vi "Get Random.vi"(7 "Func_Ext":string, 8 "에러 입력":errorcluster caption="에러 입력(에러 없음)", 10 "분해능":string caption="분해능(우선적용)", 11 "Meas":refnum<vi>[](array[refnum])) -> (0 "에러 출력":errorcluster, 3 "Meas out":refnum<vi>[](array[refnum]))   [LabVIEW 2020]
uses:
  Controls/Cmd_Var Data IO.ctl
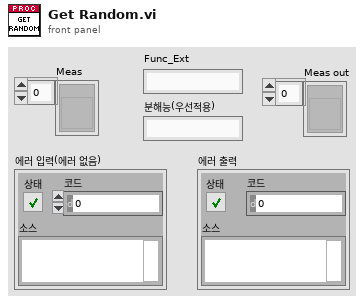
[diagram p1: front panel]
types:
  T1 = typedef "Cmd_Var Data IO.ctl" = enum16{"Condition", "Condition Default", "Condition_Temp", "Resolution", "Resolution Default", "Resolution Old", "Spec", "Spec Default", "Spec Old", "Spec Temp", "Result", "Result2", "Result3", "Result_Temp", "Result_ADJ", "Result_ADJ2", "STD1", "STD2", "STD3", "STD4", "STD5", "STD Temp", "CMC", "CMC Default"}
  T2 = enum8{"Enabled", "Disabled", "Disabled and Grayed Out"}
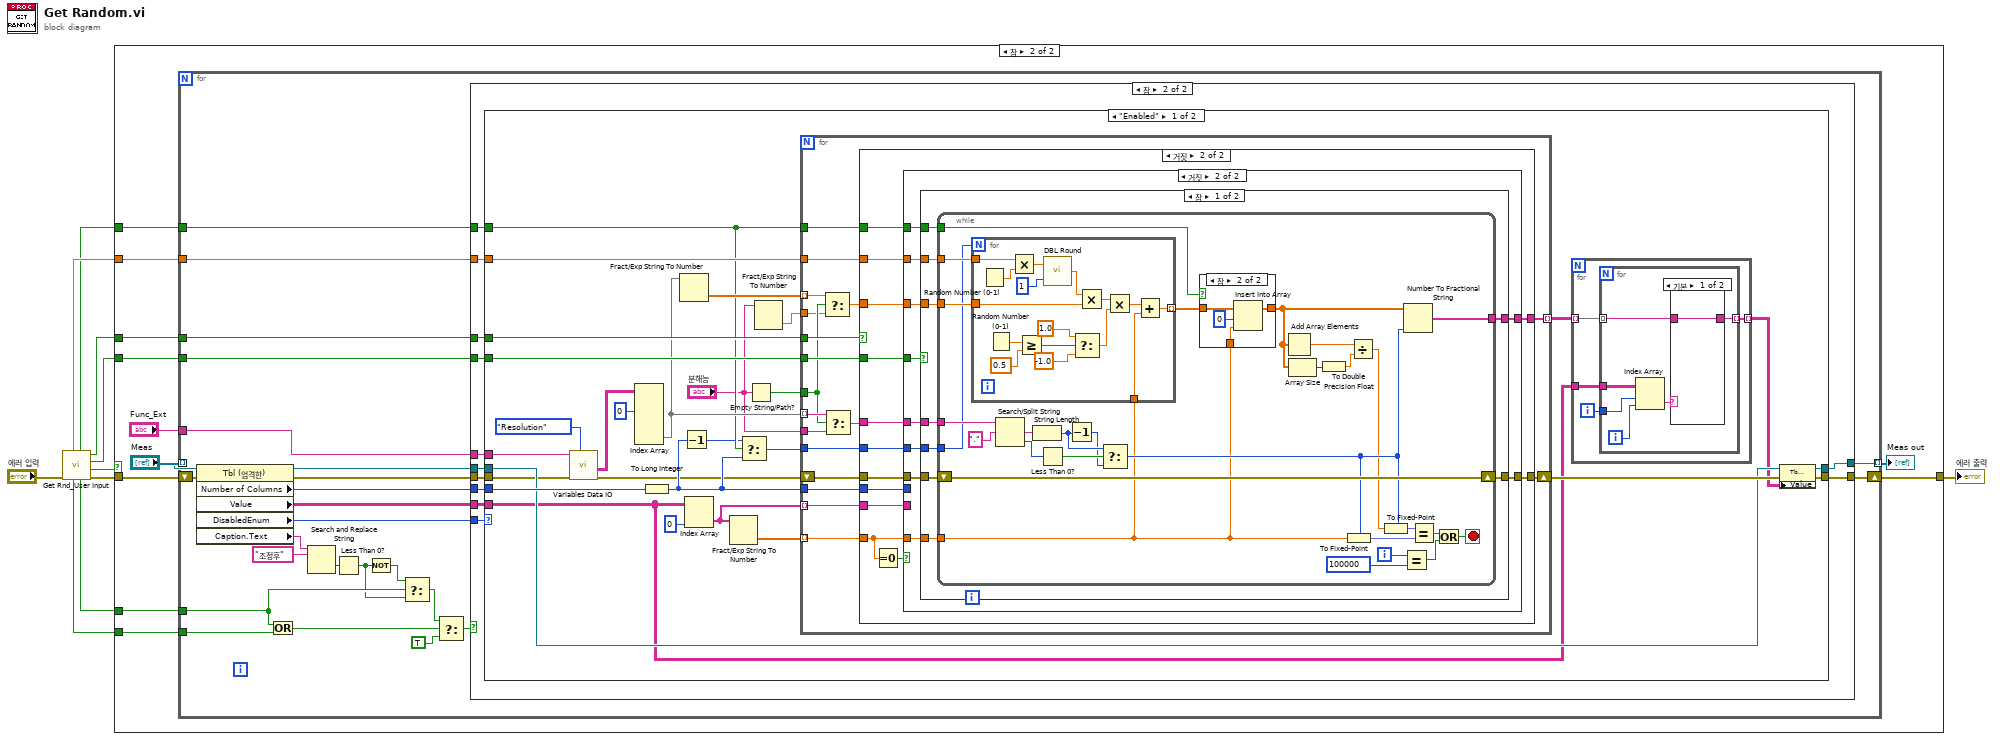
[diagram p0: block diagram]
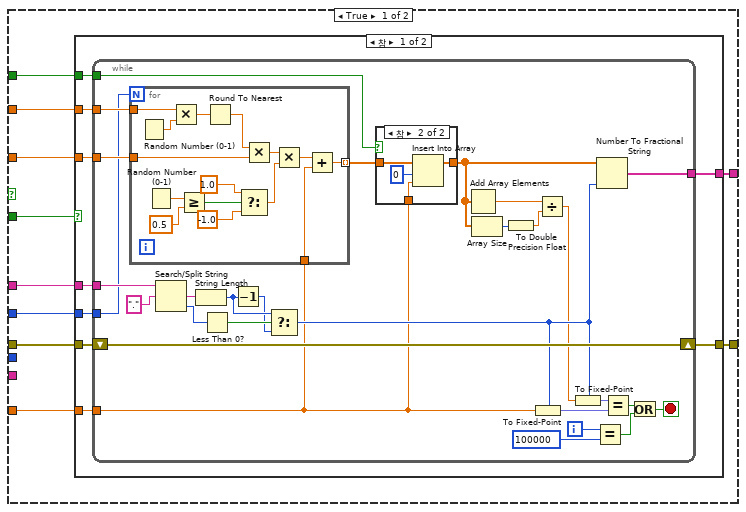
[diagram p5: hidden frame]
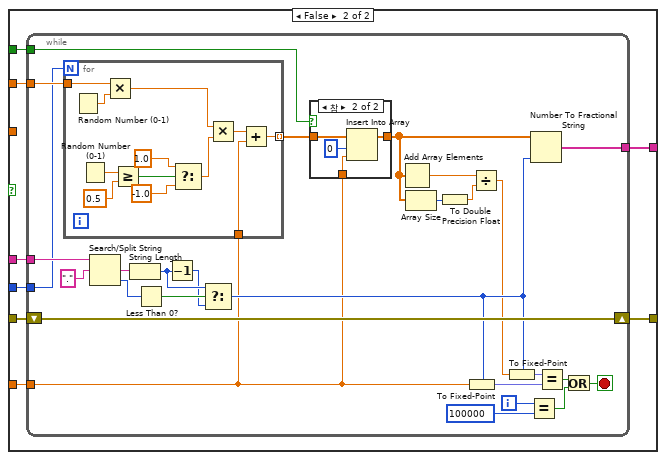
[diagram p7: hidden frame]
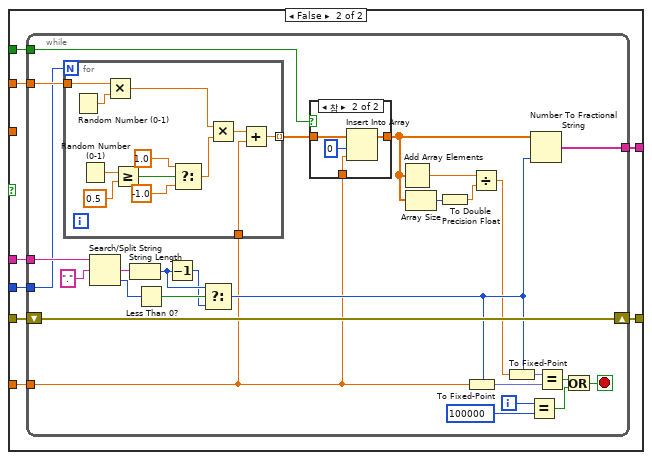
[diagram p11: hidden frame]
diagram:
  n1 = call "Get Rnd_User Input.vi"("error in"="에러 입력") -> ("error out"=w8:errorcluster, "변경?"=w7:bool, "분해능 기준?"=w4:bool, "0점 포함?"=w5:bool, "조정후?"=w1:bool, "1열 제외?"=w3:bool, "조정전?"=w2:bool, "변화량"=w6:dbl)  [unwired: 3 in]
  n2 = case shown="참" w7 {
    tunnel: [w11 w22] -> w10
    tunnel: w8 -> [w11 w19]
    tunnel: w6 -> [_ w18]
    tunnel: w5 -> [_ w17]
    tunnel: w4 -> [_ w16]
    tunnel: w3 -> [_ w15]
    tunnel: w2 -> [_ w13]
    tunnel: w1 -> [_ w12]
    frame False {
    }
    frame True {
      n3 = for {
        tunnel: "Meas" -> [w47] mode=indexing
        shift-right: [w44] -> w22
        shift-left: w19 -> [w37]
        tunnel: "Func_Ext" -> [w40]
        tunnel: w18 -> [w45]
        tunnel: w17 -> [w42]
        tunnel: w16 -> [w41]
        tunnel: w15 -> [w39]
        tunnel: [w34] -> w14 mode=indexing
        tunnel: w13 -> [w30]
        tunnel: w12 -> [w26]
        n4 = property on="프로퍼티 노드" class="Tbl (엄격한)"(reference=w47, error in=w37) -> (reference out=w43:refnum<vi>, error out=w36:errorcluster, "Number of Columns"=w46:u32, "Value"=w38:string[][], "DisabledEnum"=w35:T2, "Caption.Text"=w33:string)
        n5 = Or(x=w26, y=w30) -> (x .or. y?=w28:bool)
        n6 = Search and Replace String(input string=w33, search string="조정후" ("검색 문자열")) -> (offset past replacement=w27:i32)  [unwired: 6 in, 3 out]
        n7 = Less Than 0?(x=w27) -> (x < 0?=w24:bool)
        n8 = Not(x=w24) -> (.not. x?=w23:bool)
        n9 = Select(t=w23, s=w26, f=w24) -> (s? t:f=w25:bool)
        n10 = Select(t=w25, s=w28, f=TRUE) -> (s? t:f=w31:bool)
        n11 = case shown="참" w31 {
          tunnel: w46 -> [_ w61]
          tunnel: w45 -> [_ w60]
          tunnel: [w48 w59] -> w44
          tunnel: w43 -> [w49 w58]
          tunnel: w42 -> [_ w57]
          tunnel: w41 -> [_ w56]
          tunnel: w40 -> [_ w55]
          tunnel: w39 -> [_ w54]
          tunnel: w38 -> [_ w53]
          tunnel: w36 -> [w48 w52]
          tunnel: w35 -> [_ w51]
          tunnel: [w49 w50] -> w34
          frame False {
          }
          frame True {
            n12 = case shown="\"Enabled\"" w51 {
              tunnel: w61 -> [w89 _]
              tunnel: w60 -> [w83 _]
              tunnel: [w81 w379] -> w59
              tunnel: w58 -> [w80 w378]
              tunnel: w57 -> [w79 _]
              tunnel: w56 -> [w77 _]
              tunnel: w55 -> [w75 _]
              tunnel: w54 -> [w74 _]
              tunnel: w53 -> [w67 _]
              tunnel: w52 -> [w64 w379]
              tunnel: [w62 w378] -> w50
              frame "Enabled" {
                n13 = call "Variables Data IO.vi"("Select"=Cmd_Var_Data_IO."Resolution", "error in"=w64, "Func_ext"=w75) -> ("error out"=w63:errorcluster, "Data Out"=w86:string[][])  [unwired: 6 in, 1 out]
                n14 = Index Array(array=w86, index (col) #1=0 ("비활성화된 인덱스 (열)")) -> (element #3=w76:string[])  [unwired: 5 in, 2 out]
                n15 = To Long Integer(number=w89) -> (32bit integer=w72:i32)
                n16 = Fract/Exp String To Number(string=w76) -> (number=w85:dbl[])  [unwired: 3 in, 1 out]
                n17 = Decrement(x=w72) -> (x-1=w73:i32)
                n18 = Index Array(array=w67, index (col)=0 ("비활성화된 인덱스 (열)")) -> (element=w78:string[])  [unwired: 1 in]
                n19 = Fract/Exp String To Number(string=w78) -> (number=w88:dbl[])  [unwired: 3 in, 1 out]
                n20 = Select(t=w73, s=w74, f=w72) -> (s? t:f=w71:i32)
                n21 = Empty String/Path?(string/path="분해능") -> (empty?=w70:bool)
                n22 = Fract/Exp String To Number(string="분해능") -> (number=w68:dbl)  [unwired: 3 in, 1 out]
                n23 = for {
                  tunnel: w88 -> [w119] mode=indexing
                  tunnel: w72 -> [w120]
                  shift-right: [w117] -> w82
                  shift-left: w63 -> [w118]
                  tunnel: w85 -> [w105] mode=indexing
                  tunnel: w76 -> [w109] mode=indexing
                  tunnel: w83 -> [w116]
                  tunnel: [w115] -> w66 mode=indexing
                  tunnel: w79 -> [w114]
                  tunnel: w78 -> [w113] mode=indexing
                  tunnel: w77 -> [w112]
                  tunnel: w74 -> [w111]
                  tunnel: w71 -> [w110]
                  tunnel: w70 -> [w104]
                  tunnel: "분해능" -> [w107]
                  tunnel: w68 -> [w103]
                  n24 = Select(t=w105, s=w104, f=w103) -> (s? t:f=w106:dbl)
                  n25 = Select(t=w109, s=w104, f=w107) -> (s? t:f=w108:string)
                  n26 = case shown="거짓" w114 {
                    tunnel: w120 -> [_ w252]
                    tunnel: w119 -> [w123 w243]
                    tunnel: w106 -> [w127 w246]
                    tunnel: w108 -> [w125 w251]
                    tunnel: w118 -> [w124 w250]
                    tunnel: [w129 w249] -> w117
                    tunnel: w116 -> [w128 w248]
                    tunnel: [w130 w247] -> w115
                    tunnel: w113 -> [_ w244]
                    tunnel: w112 -> [w126 w242]
                    tunnel: w111 -> [w121 w241]
                    tunnel: w110 -> [w122 w240]
                    frame True {
                      n27 = case shown="참" w126 {
                        tunnel: w123 -> [w139 w195]
                        tunnel: w127 -> [w138 _]
                        tunnel: w125 -> [w137 w194]
                        tunnel: w124 -> [w136 w193]
                        tunnel: [w135 w192] -> w129
                        tunnel: w128 -> [w134 w191]
                        tunnel: [w133 w190] -> w130
                        tunnel: w122 -> [w132 w189]
                        tunnel: w121 -> [w131 w188]
                        frame True {
                          n28 = while {
                            tunnel: w139 -> [w143]
                            tunnel: w138 -> [w167]
                            tunnel: w137 -> [w166]
                            shift-right: [w163] -> w135
                            shift-left: w136 -> [w163]
                            tunnel: w134 -> [w151]
                            tunnel: [w149] -> w133
                            tunnel: w132 -> [w144]
                            tunnel: w131 -> [w140]
                            i -> [w165]
                            stop <- w158 stop-if-true
                            n29 = for {
                              N: w144 -> [_]
                              tunnel: w143 -> [w180]
                              tunnel: w167 -> [w178]
                              tunnel: [w179] -> w141 mode=indexing
                              tunnel: w151 -> [w174]
                              n30 = Random Number (0-1)() -> (number: 0 to 1=w175:dbl)
                              n31 = Random Number (0-1)() -> (number: 0 to 1=w187:dbl)
                              n32 = Multiply(x=w174, y=w175) -> (x*y=w176:dbl)
                              n33 = Greater Or Equal?(x=w187, y=0.5) -> (x >= y?=w185:bool)
                              n34 = Round To Nearest(number=w176) -> (nearest integer value=w173:dbl)
                              n35 = Select(t=1.0, s=w185, f=-1.0) -> (s? t:f=w182:dbl)
                              n36 = Multiply(x=w173, y=w178) -> (x*y=w177:dbl)
                              n37 = Multiply(x=w177, y=w182) -> (x*y=w181:dbl)
                              n38 = Add(x=w181, y=w180) -> (x+y=w179:dbl)
                            }
                            n39 = Search/Split String(string=w166, search string/char (-)="." ("검색 문자열/문자 (-)")) -> (match + rest of string=w157:string, offset of match=w155:i32)  [unwired: 1 in, 1 out]
                            n40 = String Length(string=w157) -> (length=w153:i32)
                            n41 = Less Than 0?(x=w155) -> (x < 0?=w154:bool)
                            n42 = Decrement(x=w153) -> (x-1=w152:i32)
                            n43 = Select(t=w153, s=w154, f=w152) -> (s? t:f=w150:i32)
                            n44 = case shown="참" w140 {
                              tunnel: w141 -> [w168 w172]
                              tunnel: w143 -> [_ w170]
                              tunnel: [w168 w169] -> w142
                              frame False {
                              }
                              frame True {
                                n45 = Insert Into Array(array=w172, index=0 ("인덱스"), new element=w170) -> (w169:dbl[])
                              }
                            }
                            n46 = Add Array Elements(numeric array=w142) -> (sum=w148:dbl)
                            n47 = Array Size(array=w142) -> (size(s)=w147:i32)
                            n48 = To Double Precision Float(number=w147) -> (double precision float=w146:dbl)
                            n49 = To Fixed-Point(fixed-point type=w150, number=w143) -> (fixed-point=w161:fxp<+/-,32,32>)
                            n50 = Divide(x=w148, y=w146) -> (x/y=w145:dbl)
                            n51 = To Fixed-Point(fixed-point type=w150, number=w145) -> (fixed-point=w162:fxp<+/-,32,32>)
                            n52 = Equal?(x=w165, y=100000) -> (x = y?=w159:bool)
                            n53 = Number To Fractional String(number=w142, precision (6)=w150) -> (F-format string=w149:string[])  [unwired: 2 in]
                            n54 = Equal?(x=w162, y=w161) -> (x = y?=w160:bool)
                            n55 = Or(x=w160, y=w159) -> (x .or. y?=w158:bool)
                          }
                        }
                        frame False {
                          n56 = while {
                            tunnel: w195 -> [w203]
                            tunnel: w194 -> [w222]
                            shift-right: [w219] -> w192
                            shift-left: w193 -> [w219]
                            tunnel: w191 -> [w207]
                            tunnel: [w204] -> w190
                            tunnel: w189 -> [w197]
                            tunnel: w188 -> [w196]
                            i -> [w221]
                            stop <- w214 stop-if-true
                            n57 = for {
                              N: w197 -> [_]
                              tunnel: w203 -> [w238]
                              tunnel: [w237] -> w206 mode=indexing
                              tunnel: w207 -> [w229]
                              n58 = Random Number (0-1)() -> (number: 0 to 1=w236:dbl)
                              n59 = Random Number (0-1)() -> (number: 0 to 1=w235:dbl)
                              n60 = Multiply(x=w229, y=w236) -> (x*y=w228:dbl)
                              n61 = Greater Or Equal?(x=w235, y=0.5) -> (x >= y?=w234:bool)
                              n62 = Select(t=1.0, s=w234, f=-1.0) -> (s? t:f=w232:dbl)
                              n63 = Multiply(x=w228, y=w232) -> (x*y=w239:dbl)
                              n64 = Add(x=w239, y=w238) -> (x+y=w237:dbl)
                            }
                            n65 = Search/Split String(string=w222, search string/char (-)="." ("검색 문자열/문자 (-)")) -> (match + rest of string=w213:string, offset of match=w211:i32)  [unwired: 1 in, 1 out]
                            n66 = String Length(string=w213) -> (length=w209:i32)
                            n67 = Less Than 0?(x=w211) -> (x < 0?=w210:bool)
                            n68 = Decrement(x=w209) -> (x-1=w208:i32)
                            n69 = Select(t=w209, s=w210, f=w208) -> (s? t:f=w205:i32)
                            n70 = case shown="참" w196 {
                              tunnel: w206 -> [w223 w227]
                              tunnel: w203 -> [_ w225]
                              tunnel: [w223 w224] -> w199
                              frame False {
                              }
                              frame True {
                                n71 = Insert Into Array(array=w227, index=0 ("인덱스"), new element=w225) -> (w224:dbl[])
                              }
                            }
                            n72 = Add Array Elements(numeric array=w199) -> (sum=w202:dbl)
                            n73 = Array Size(array=w199) -> (size(s)=w201:i32)
                            n74 = To Double Precision Float(number=w201) -> (double precision float=w200:dbl)
                            n75 = To Fixed-Point(fixed-point type=w205, number=w203) -> (fixed-point=w217:fxp<+/-,32,32>)
                            n76 = Divide(x=w202, y=w200) -> (x/y=w198:dbl)
                            n77 = To Fixed-Point(fixed-point type=w205, number=w198) -> (fixed-point=w218:fxp<+/-,32,32>)
                            n78 = Equal?(x=w221, y=100000) -> (x = y?=w215:bool)
                            n79 = Number To Fractional String(number=w199, precision (6)=w205) -> (F-format string=w204:string[])  [unwired: 2 in]
                            n80 = Equal?(x=w218, y=w217) -> (x = y?=w216:bool)
                            n81 = Or(x=w216, y=w215) -> (x .or. y?=w214:bool)
                          }
                        }
                      }
                    }
                    frame False {
                      n82 = Equal To 0?(x=w243) -> (x = 0?=w245:bool)
                      n83 = case shown="거짓" w245 {
                        tunnel: w252 -> [w255 _]
                        tunnel: w243 -> [_ w267]
                        tunnel: w246 -> [_ w266]
                        tunnel: w251 -> [_ w265]
                        tunnel: w250 -> [w256 w264]
                        tunnel: [w256 w263] -> w249
                        tunnel: w248 -> [_ w262]
                        tunnel: [w254 w261] -> w247
                        tunnel: w244 -> [w253 _]
                        tunnel: w242 -> [_ w260]
                        tunnel: w241 -> [_ w259]
                        tunnel: w240 -> [_ w258]
                        frame True {
                          n84 = for {
                            N: w255 -> [_]
                            tunnel: w253 -> [w257]
                            tunnel: [w257] -> w254 mode=indexing
                          }
                        }
                        frame False {
                          n85 = case shown="참" w260 {
                            tunnel: w267 -> [w276 w333]
                            tunnel: w266 -> [w275 _]
                            tunnel: w265 -> [w274 w332]
                            tunnel: w264 -> [w273 w331]
                            tunnel: [w272 w330] -> w263
                            tunnel: w262 -> [w271 w329]
                            tunnel: [w270 w328] -> w261
                            tunnel: w259 -> [w269 w326]
                            tunnel: w258 -> [w268 w327]
                            frame True {
                              n86 = while {
                                tunnel: w276 -> [w279]
                                tunnel: w275 -> [w304]
                                tunnel: w274 -> [w303]
                                shift-right: [w300] -> w272
                                shift-left: w273 -> [w300]
                                tunnel: w271 -> [w288]
                                tunnel: [w286] -> w270
                                tunnel: w269 -> [w277]
                                tunnel: w268 -> [w281]
                                i -> [w302]
                                stop <- w295 stop-if-true
                                n87 = for {
                                N: w281 -> [_]
                                tunnel: w279 -> [w318]
                                tunnel: w304 -> [w314]
                                tunnel: [w317] -> w280 mode=indexing
                                tunnel: w288 -> [w315]
                                n88 = Random Number (0-1)() -> (number: 0 to 1=w316:dbl)
                                n89 = Random Number (0-1)() -> (number: 0 to 1=w325:dbl)
                                n90 = Multiply(x=w315, y=w316) -> (x*y=w312:dbl)
                                n91 = Greater Or Equal?(x=w325, y=0.5) -> (x >= y?=w323:bool)
                                n92 = call "DBL Round.vi"("반올림자리수"=1 ("자리수"), "DBL in"=w312) -> ("DBL out"=w311:dbl)  [unwired: 1 in]
                                n93 = Select(t=1.0, s=w323, f=-1.0) -> (s? t:f=w320:dbl)
                                n94 = Multiply(x=w311, y=w314) -> (x*y=w313:dbl)
                                n95 = Multiply(x=w313, y=w320) -> (x*y=w319:dbl)
                                n96 = Add(x=w319, y=w318) -> (x+y=w317:dbl)
                                }
                                n97 = Search/Split String(string=w303, search string/char (-)="." ("검색 문자열/문자 (-)")) -> (match + rest of string=w294:string, offset of match=w292:i32)  [unwired: 1 in, 1 out]
                                n98 = String Length(string=w294) -> (length=w290:i32)
                                n99 = Less Than 0?(x=w292) -> (x < 0?=w291:bool)
                                n100 = Decrement(x=w290) -> (x-1=w289:i32)
                                n101 = Select(t=w290, s=w291, f=w289) -> (s? t:f=w287:i32)
                                n102 = case shown="참" w277 {
                                tunnel: w280 -> [w305 w309]
                                tunnel: w279 -> [_ w307]
                                tunnel: [w305 w306] -> w278
                                frame False {
                                }
                                frame True {
                                n103 = Insert Into Array(array=w309, index=0 ("인덱스"), new element=w307) -> (w306:dbl[])
                                }
                                }
                                n104 = Add Array Elements(numeric array=w278) -> (sum=w285:dbl)
                                n105 = Array Size(array=w278) -> (size(s)=w284:i32)
                                n106 = To Double Precision Float(number=w284) -> (double precision float=w283:dbl)
                                n107 = To Fixed-Point(fixed-point type=w287, number=w279) -> (fixed-point=w298:fxp<+/-,32,32>)
                                n108 = Divide(x=w285, y=w283) -> (x/y=w282:dbl)
                                n109 = To Fixed-Point(fixed-point type=w287, number=w282) -> (fixed-point=w299:fxp<+/-,32,32>)
                                n110 = Equal?(x=w302, y=100000) -> (x = y?=w296:bool)
                                n111 = Number To Fractional String(number=w278, precision (6)=w287) -> (F-format string=w286:string[])  [unwired: 2 in]
                                n112 = Equal?(x=w299, y=w298) -> (x = y?=w297:bool)
                                n113 = Or(x=w297, y=w296) -> (x .or. y?=w295:bool)
                              }
                            }
                            frame False {
                              n114 = while {
                                tunnel: w333 -> [w336]
                                tunnel: w332 -> [w360]
                                shift-right: [w357] -> w330
                                shift-left: w331 -> [w357]
                                tunnel: w329 -> [w345]
                                tunnel: [w343] -> w328
                                tunnel: w327 -> [w338]
                                tunnel: w326 -> [w334]
                                i -> [w359]
                                stop <- w352 stop-if-true
                                n115 = for {
                                N: w338 -> [_]
                                tunnel: w336 -> [w376]
                                tunnel: [w375] -> w337 mode=indexing
                                tunnel: w345 -> [w367]
                                n116 = Random Number (0-1)() -> (number: 0 to 1=w374:dbl)
                                n117 = Random Number (0-1)() -> (number: 0 to 1=w373:dbl)
                                n118 = Multiply(x=w367, y=w374) -> (x*y=w366:dbl)
                                n119 = Greater Or Equal?(x=w373, y=0.5) -> (x >= y?=w372:bool)
                                n120 = Select(t=1.0, s=w372, f=-1.0) -> (s? t:f=w370:dbl)
                                n121 = Multiply(x=w366, y=w370) -> (x*y=w377:dbl)
                                n122 = Add(x=w377, y=w376) -> (x+y=w375:dbl)
                                }
                                n123 = Search/Split String(string=w360, search string/char (-)="." ("검색 문자열/문자 (-)")) -> (match + rest of string=w351:string, offset of match=w349:i32)  [unwired: 1 in, 1 out]
                                n124 = String Length(string=w351) -> (length=w347:i32)
                                n125 = Less Than 0?(x=w349) -> (x < 0?=w348:bool)
                                n126 = Decrement(x=w347) -> (x-1=w346:i32)
                                n127 = Select(t=w347, s=w348, f=w346) -> (s? t:f=w344:i32)
                                n128 = case shown="참" w334 {
                                tunnel: w337 -> [w361 w365]
                                tunnel: w336 -> [_ w363]
                                tunnel: [w361 w362] -> w335
                                frame False {
                                }
                                frame True {
                                n129 = Insert Into Array(array=w365, index=0 ("인덱스"), new element=w363) -> (w362:dbl[])
                                }
                                }
                                n130 = Add Array Elements(numeric array=w335) -> (sum=w342:dbl)
                                n131 = Array Size(array=w335) -> (size(s)=w341:i32)
                                n132 = To Double Precision Float(number=w341) -> (double precision float=w340:dbl)
                                n133 = To Fixed-Point(fixed-point type=w344, number=w336) -> (fixed-point=w355:fxp<+/-,32,32>)
                                n134 = Divide(x=w342, y=w340) -> (x/y=w339:dbl)
                                n135 = To Fixed-Point(fixed-point type=w344, number=w339) -> (fixed-point=w356:fxp<+/-,32,32>)
                                n136 = Equal?(x=w359, y=100000) -> (x = y?=w353:bool)
                                n137 = Number To Fractional String(number=w335, precision (6)=w344) -> (F-format string=w343:string[])  [unwired: 2 in]
                                n138 = Equal?(x=w356, y=w355) -> (x = y?=w354:bool)
                                n139 = Or(x=w354, y=w353) -> (x .or. y?=w352:bool)
                              }
                            }
                          }
                        }
                      }
                    }
                  }
                }
                n140 = for {
                  tunnel: w67 -> [w94]
                  tunnel: w66 -> [w93] mode=indexing
                  tunnel: [w91] -> w65 mode=indexing
                  i -> [w92]
                  n141 = for {
                    tunnel: w94 -> [w100]
                    tunnel: w93 -> [w96] mode=indexing
                    tunnel: w92 -> [w99]
                    tunnel: [w95] -> w91 mode=indexing
                    i -> [w98]
                    n142 = Index Array(array=w100, index (row)=w99, index (col)=w98) -> (element=w97:string)
                    n143 = case shown="기본" w97 {
                      selector: w97 -> [_ w102]
                      tunnel: w96 -> [w101 _]
                      tunnel: [w101 w102] -> w95
                      frame Default {
                      }
                      frame "ⅹ" {
                      }
                    }
                  }
                }
                n144 = property on="프로퍼티 노드" class="Tbl (엄격한)"(reference=w80, error in=w82, "Value"=w65) -> (reference out=w62:refnum<vi>, error out=w81:errorcluster)
              }
              frame Default {
              }
            }
          }
        }
      }
      "Meas out" <- w14
    }
  }
  "에러 출력" <- w10
